vi "test_output_mixing_scale.vi"() -> ()   [LabVIEW 2013]
panel:
  out "Z":i16
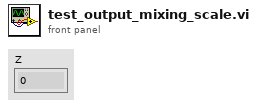
[diagram p1: front panel]
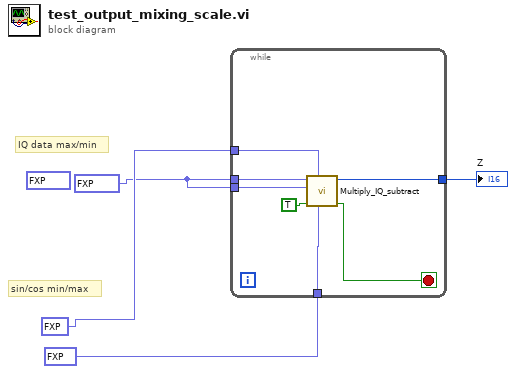
[diagram p0: block diagram]
diagram:
  w1 = fxp<+/-,16,14> 2697.25 ("max value")
  (unwired) fxp<+/-,16,14> -2698.5 ("min value")
  # "IQ data max/min"
  # "sin/cos min/max"
  n1 = while {
    tunnel: w1 -> [w11]
    tunnel: w1 -> [w10]
    tunnel: fxp<+/-,16,0> -0.25 ("min value") -> [w9]
    tunnel: fxp<+/-,16,0> 0.25 ("max value") -> [w8]
    tunnel: [w7] -> w2
    stop <- w5 stop-if-true
    n2 = call "Multiply_IQ_subtract.vi"("Sin"=w9, "Cos"=w8, "input valid"=TRUE, "Q"=w10, "I"=w11) -> ("output valid"=w5:bool, "Z"=w7:i16)  [unwired: 5 in]
  }
  "Z" <- w2
